vi "ExpCreateMatlabService.vi"(11 "envpath":path) -> ()   [LabVIEW 2017]
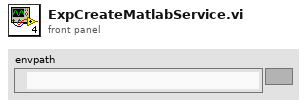
[diagram p1: front panel]
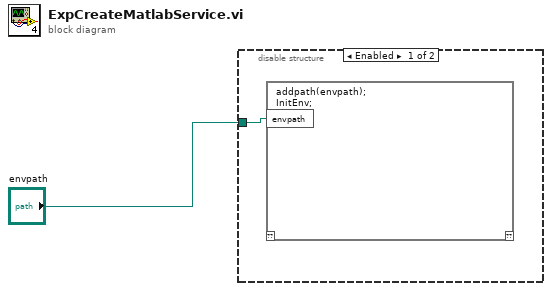
[diagram p0: block diagram]
diagram:
  n1 = disable-structure shown="Enabled" {
    disable-tunnel: "envpath" -> [w2 _]
    frame Enabled {
      n2 = script code="addpath(envpath);\nInitEnv;"("envpath"=w2) -> ()  [unwired: 1 in, 1 out]
    }
    frame Disabled {
    }
  }
